vi "Read Single Analog Channel.vi"(8 "error in (no error)":errorcluster, 9 "Channel":T1(ring), 10 "Voltage Data":bool=TRUE, 11 "VISA resource name":refnum<visa-resource-name>) -> (0 "error out":errorcluster, 2 "Channel Data":dbl, 3 "VISA resource name":refnum<visa-resource-name>)   [LabVIEW 2020, in "BDAQ-6104.lvlib"]
uses:
  <instrlib>/BDAQ-6104/BDAQ-6104.lvlib
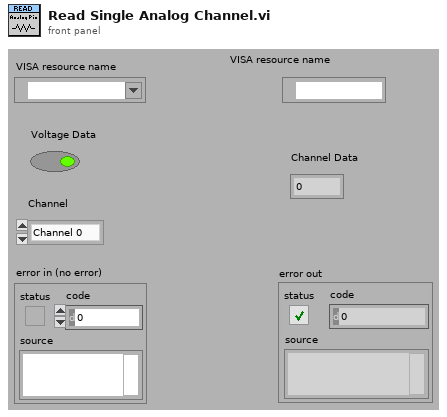
[diagram p1: front panel]
types:
  T1 = enum16{"Channel 0", "Channel 1", "Channel 2", "Channel 3", "Channel 4", "Channel 5"}
  T2 = cluster{"AIO-0":dbl, "AIO-1":dbl, "AIO-2":dbl, "AIO-3":dbl, "AIO-4":dbl, "AIO-5":dbl}
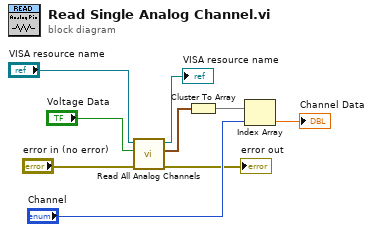
[diagram p0: block diagram]
diagram:
  n1 = call <instrlib>:"Read All Analog Channels.vi"("error in"="error in (no error)", "Voltage Data"="Voltage Data", "VISA resource name"="VISA resource name") -> ("error out"=→"error out":errorcluster, "Analog output cluster"=w6:T2, "VISA resource name out"=→"VISA resource name":refnum<visa-resource-name>)  [unwired: 5 in]
  n2 = Cluster To Array(cluster=w6) -> (array=w5:dbl[])
  n3 = Index Array(array=w5, index="Channel") -> (element=→"Channel Data":dbl)
